vi "CONTROLLER.vi"(8 "error in (no error)":errorcluster, 11 "control\ncluster":T1) -> (0 "error out":errorcluster, 3 "control\ncluster out":T1)   [LabVIEW 2023]
uses:
  Global odometry.vi
  ctrl defs/ctrl controllers.ctl
panel:
  out "set\nLOCKs":bool=TRUE
  out "Buttons":bool[](array[boolean])
  out "POVs":i16[](array[numeric])
  in  "axis scale":dbl=0.7 format="%#_13g"
  out "Axes":dbl[](array[numeric])
  in  "axis dead band":dbl=0.025 format="%#_13g"
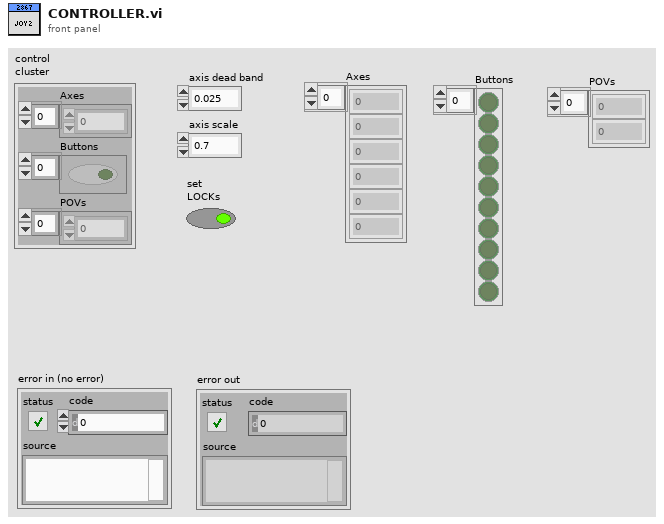
[diagram p1: front panel]
types:
  T1 = typedef "ctrl controllers.ctl" = cluster{"Axes":dbl[], "Buttons":bool[], "POVs":i16[]}
  T2 = cluster{"LEFT ARM":cluster{"VBus%":dbl, "LOCK?":bool, "LOCKED":bool}, "RIGHT ARM":cluster{"VBus%":dbl, "LOCK?":bool, "LOCKED":bool}}
  T3 = cluster{"VBus%":dbl, "LOCK?":bool, "LOCKED":bool}
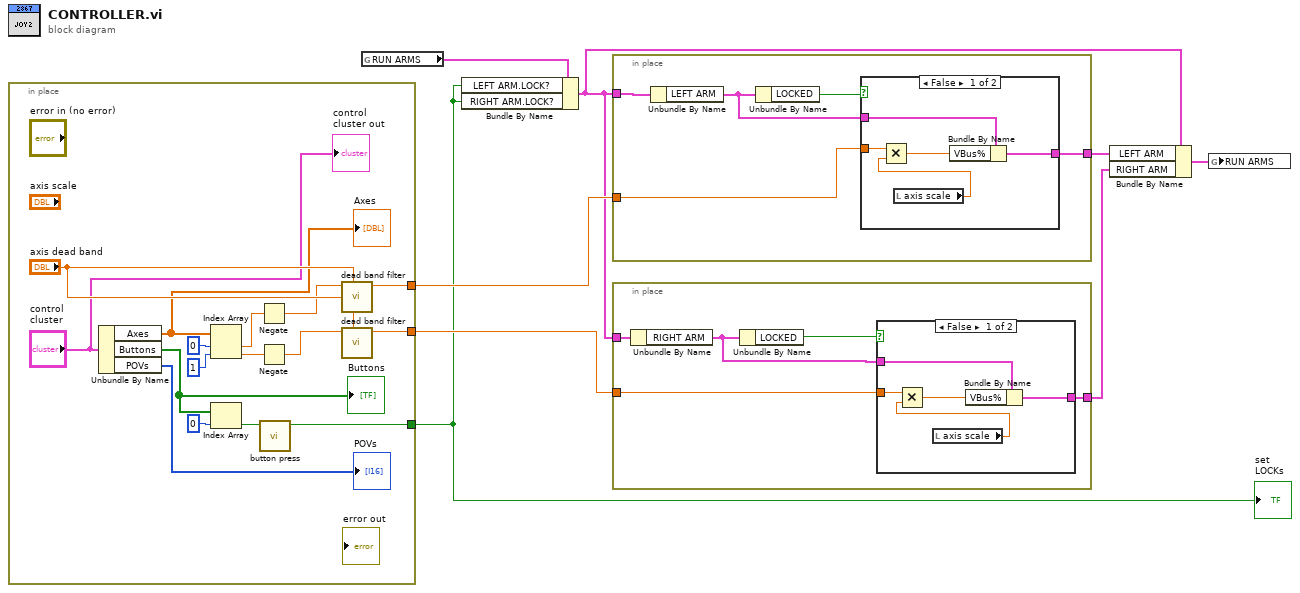
[diagram p0: block diagram]
diagram:
  n1 = in-place {
    in-place-border: [w17] -> w8
    in-place-border: [w16] -> w7
    in-place-border: [w9] -> w2
    n2 = Unbundle By Name("control\ncluster") -> ("Axes"=w14:dbl[], "Buttons"=w12:bool[], "POVs"=→"POVs":i16[])
    "Axes" <- w14
    "Buttons" <- w12
    n3 = Index Array(array=w14, index #1=0 ("index"), index #2=1 ("index")) -> (element #1=w21:dbl, element #2=w20:dbl)
    n4 = Index Array(array=w12, index=0) -> (element=w11:bool)
    n5 = Negate(x=w21) -> (-x=w19:dbl)
    n6 = Negate(x=w20) -> (-x=w18:dbl)
    n7 = call "button press.vi"("button IN"=w11) -> ("Button Pressed?"=w9:bool)  [unwired: 10 in]
    n8 = call "dead band filter.vi"("deadband"="axis dead band", "input"=w19) -> ("output"=w17:dbl)  [unwired: 9 in]
    n9 = call "dead band filter.vi"("deadband"="axis dead band", "input"=w18) -> ("output"=w16:dbl)  [unwired: 9 in]
    "control\ncluster out" <- "control\ncluster"
  }
  "set\nLOCKs" <- w2
  n10 = global read "Global odometry.vi" "RUN ARMS"() -> (w3:T2)
  n11 = Bundle By Name(cluster=w3, "LEFT ARM.LOCK?"=w2, "RIGHT ARM.LOCK?"=w2) -> (w1:T2)
  n12 = in-place {
    in-place-border: w8 -> [w29]
    in-place-border: [w26] -> w5
    in-place-border: w1 -> [w25]
    n13 = Unbundle By Name(w25) -> ("LEFT ARM"=w27:T3)
    n14 = Unbundle By Name(w27) -> ("LOCKED"=w28:bool)
    n15 = case shown="False" w28 {
      tunnel: w29 -> [w34 _]
      tunnel: [w33 w35] -> w26
      tunnel: w27 -> [w32 w35]
      frame False {
        n16 = local read "axis scale"() -> (w30:dbl)
        n17 = Multiply(x=w34, y=w30) -> (x*y=w31:dbl)
        n18 = Bundle By Name(cluster=w32, "VBus%"=w31) -> (w33:T3)
      }
      frame True {
      }
    }
  }
  n19 = in-place {
    in-place-border: w7 -> [w38]
    in-place-border: [w37] -> w4
    in-place-border: w1 -> [w36]
    n20 = Unbundle By Name(w36) -> ("RIGHT ARM"=w40:T3)
    n21 = Unbundle By Name(w40) -> ("LOCKED"=w39:bool)
    n22 = case shown="False" w39 {
      tunnel: w38 -> [w44 _]
      tunnel: [w43 w46] -> w37
      tunnel: w40 -> [w42 w46]
      frame False {
        n23 = local read "axis scale"() -> (w41:dbl)
        n24 = Multiply(x=w44, y=w41) -> (x*y=w45:dbl)
        n25 = Bundle By Name(cluster=w42, "VBus%"=w45) -> (w43:T3)
      }
      frame True {
      }
    }
  }
  n26 = Bundle By Name(cluster=w1, "LEFT ARM"=w5, "RIGHT ARM"=w4) -> (w6:T2)
  n27 = global write "Global odometry.vi" "RUN ARMS"(w6) -> ()
